vi "Power Rider Demo .vi"() -> ()   [LabVIEW 2017]
panel:
  out "Current [A]":sgl
  out "Vout [V]":sgl
  out "Switch":bool
  out "Status":u8(ring) items=["OFF", "ON", "ERROR", "FOREVER OFF"]
  out "Vin [V]":sgl
  out "Trip Type":u16(ring)=2 items=["Not tripped", "SW Tripped", "Hard Short", "MAX SW Tripped"]
  in  "ChannelNum":i32=1
  out "Unit P_N":string
  out "SW Version":string
  in  "dstAdd":u8=16
  in  "ID address":u8=85
  out "dllVersion":string
  # "Power Rider Demo"
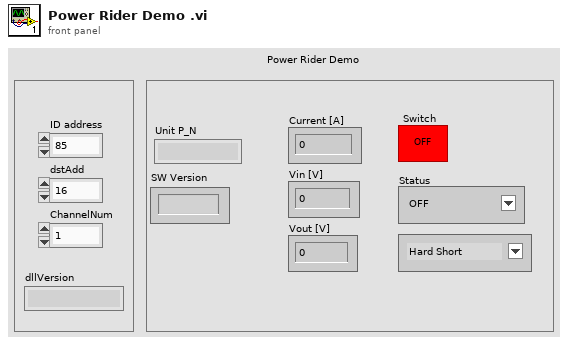
[diagram p1: front panel]
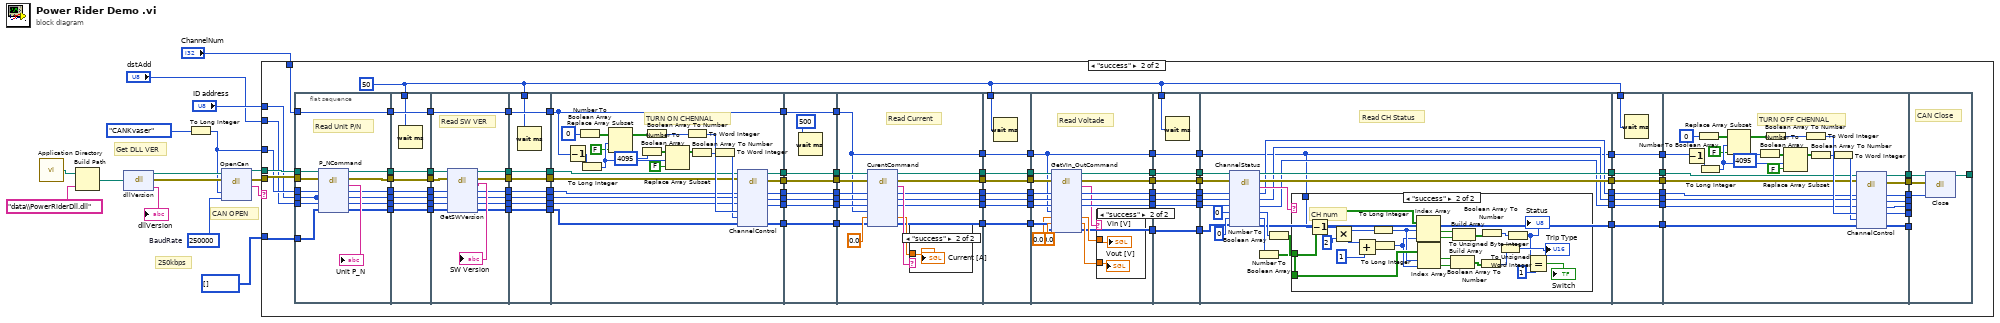
[diagram p0: block diagram]
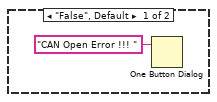
[diagram p2: hidden frame]
diagram:
  w12 = u32 250000  # BaudRate
  # "CAN OPEN"
  # "Get DLL VER"
  # "250kbps"
  n1 = call <vilib>:"Application Directory.vi"() -> ("Application Directory"=w16:path)
  n2 = Build Path(base path=w16, name or relative path="data\\PowerRiderDll.dll") -> (appended path=w14:path)
  n3 = dll-call lib="C:/Projects/Fuse/PowerRider-DLL-GUI/PRDLL/Labview/data/PowerRiderDll.dll" fn="dllVersion"(path in=w14) -> (path out=w11:path, error out=w10:errorcluster, "return type"=→"dllVersion":string)  [unwired: 2 in]
  n4 = To Long Integer(number=enum32{"None", "CANalystII", "UDP", "CANKvaser"}."CANKvaser") -> (32bit integer=w5:i32)
  n5 = dll-call lib="C:/Projects/Fuse/PowerRider-DLL-GUI/PRDLL/Labview/data/PowerRiderDll.dll" fn="OpenCan"(path in=w11, error in=w10, "type"=w5, "BaudRate"=w12) -> (path out=w9:path, error out=w8:errorcluster, "return type"=w7:string)  [unwired: 3 in]
  n6 = case shown="\"success\"" w7 {
    tunnel: w9 -> [_ w111]
    tunnel: w8 -> [_ w110]
    tunnel: w5 -> [_ w109]
    tunnel: "ID address" -> [_ w108]
    tunnel: "dstAdd" -> [_ w107]
    tunnel: u8[] [] ("PsNetwork") -> [_ w112]
    tunnel: "ChannelNum" -> [_ w106]
    frame "False", Default {
      n7 = One Button Dialog(message="CAN Open Error !!! ") -> ()  [unwired: 1 in, 1 out]
    }
    frame "success" {
      w18 = u32 50 ("milliseconds to wait")
      n8 = flat-sequence {
        tunnel: w106 -> [w130]
        tunnel: [w130] -> w113
        tunnel: w112 -> [w128]
        tunnel: w111 -> [w127]
        tunnel: w110 -> [w126]
        tunnel: w109 -> [w125]
        tunnel: [w124] -> _
        tunnel: w108 -> [w124]
        tunnel: w107 -> [w123]
        tunnel: [w122] -> w104
        tunnel: [w121] -> w102
        tunnel: [w120] -> w100
        tunnel: [w119] -> w98
        tunnel: [w118] -> w96
        tunnel: [w117] -> w94
        tunnel: [w138] -> w114
        tunnel: w113 -> [w138]
        tunnel: w18 -> [w137]
        tunnel: [w136] -> w105
        tunnel: w104 -> [w136]
        tunnel: [w135] -> w103
        tunnel: w102 -> [w135]
        tunnel: [w134] -> w101
        tunnel: w100 -> [w134]
        tunnel: [w133] -> w99
        tunnel: w98 -> [w133]
        tunnel: [w132] -> w97
        tunnel: w96 -> [w132]
        tunnel: [w131] -> w95
        tunnel: w94 -> [w131]
        tunnel: [w152] -> w93
        tunnel: w114 -> [w152]
        tunnel: w105 -> [w150]
        tunnel: w103 -> [w149]
        tunnel: w101 -> [w148]
        tunnel: w99 -> [w147]
        tunnel: w97 -> [w146]
        tunnel: w95 -> [w145]
        tunnel: [w144] -> w91
        tunnel: [w143] -> w89
        tunnel: [w142] -> w87
        tunnel: [w141] -> w85
        tunnel: [w140] -> w83
        tunnel: [w139] -> w81
        tunnel: w93 -> [w160]
        tunnel: [w160] -> w92
        tunnel: w91 -> [w159]
        tunnel: [w159] -> w90
        tunnel: w89 -> [w158]
        tunnel: [w158] -> w88
        tunnel: w87 -> [w157]
        tunnel: [w157] -> w86
        tunnel: w85 -> [w156]
        tunnel: [w156] -> w84
        tunnel: w83 -> [w155]
        tunnel: [w155] -> w82
        tunnel: w81 -> [w154]
        tunnel: [w154] -> w80
        tunnel: w18 -> [w153]
        tunnel: [w174] -> w115
        tunnel: w92 -> [w174]
        tunnel: w90 -> [w173]
        tunnel: w88 -> [w172]
        tunnel: w86 -> [w171]
        tunnel: w84 -> [w170]
        tunnel: w82 -> [w169]
        tunnel: w80 -> [w168]
        tunnel: [w167] -> w78
        tunnel: [w166] -> w76
        tunnel: [w165] -> w74
        tunnel: [w164] -> w72
        tunnel: [w163] -> w70
        tunnel: [w162] -> w68
        tunnel: [w195] -> w116
        tunnel: w115 -> [w195]
        tunnel: [w193] -> w79
        tunnel: w78 -> [w193]
        tunnel: [w192] -> w77
        tunnel: w76 -> [w192]
        tunnel: [w191] -> w75
        tunnel: w74 -> [w191]
        tunnel: [w190] -> w73
        tunnel: w72 -> [w190]
        tunnel: [w189] -> w71
        tunnel: w70 -> [w189]
        tunnel: [w188] -> w69
        tunnel: w68 -> [w188]
        tunnel: [w208] -> w67
        tunnel: [w207] -> w65
        tunnel: [w206] -> w63
        tunnel: [w205] -> w61
        tunnel: [w204] -> w58
        tunnel: w116 -> [w197]
        tunnel: w79 -> [w203]
        tunnel: w77 -> [w202]
        tunnel: w75 -> [w201]
        tunnel: w73 -> [w200]
        tunnel: w71 -> [w199]
        tunnel: w69 -> [w198]
        tunnel: [w197] -> w55
        tunnel: [w196] -> w54
        tunnel: w67 -> [w220]
        tunnel: [w220] -> w66
        tunnel: w65 -> [w219]
        tunnel: [w219] -> w64
        tunnel: w63 -> [w218]
        tunnel: [w218] -> w62
        tunnel: w61 -> [w214]
        tunnel: [w214] -> w60
        tunnel: [w213] -> w59
        tunnel: w58 -> [w217]
        tunnel: [w217] -> w57
        tunnel: w18 -> [w216]
        tunnel: [w215] -> w56
        tunnel: w55 -> [w215]
        tunnel: w54 -> [w213]
        tunnel: w66 -> [w236]
        tunnel: w64 -> [w235]
        tunnel: w62 -> [w234]
        tunnel: w60 -> [w232]
        tunnel: w59 -> [w231]
        tunnel: w57 -> [w237]
        tunnel: w56 -> [w221]
        tunnel: [w230] -> w53
        tunnel: [w229] -> w52
        tunnel: [w228] -> w51
        tunnel: [w227] -> w50
        tunnel: [w226] -> w49
        tunnel: [w222] -> w48
        tunnel: [w221] -> w29
        tunnel: w53 -> [w248]
        tunnel: w52 -> [w247]
        tunnel: w51 -> [w246]
        tunnel: w50 -> [w245]
        tunnel: w49 -> [w244]
        tunnel: w48 -> [w243]
        tunnel: w18 -> [w242]
        tunnel: [w248] -> w47
        tunnel: [w247] -> w46
        tunnel: [w246] -> w45
        tunnel: [w245] -> w44
        tunnel: [w244] -> w43
        tunnel: [w243] -> w42
        tunnel: w29 -> [w241]
        tunnel: [w241] -> w28
        tunnel: w47 -> [w263]
        tunnel: w46 -> [w264]
        tunnel: w45 -> [w261]
        tunnel: w44 -> [w260]
        tunnel: w43 -> [w259]
        tunnel: w42 -> [w262]
        tunnel: [w254] -> w41
        tunnel: [w255] -> w40
        tunnel: [w253] -> w39
        tunnel: [w252] -> w38
        tunnel: [w251] -> w37
        tunnel: [w250] -> w36
        tunnel: w28 -> [w249]
        tunnel: [w249] -> w20
        tunnel: w41 -> [w298]
        tunnel: w40 -> [w297]
        tunnel: w39 -> [w296]
        tunnel: w38 -> [w295]
        tunnel: w37 -> [w294]
        tunnel: w36 -> [w293]
        tunnel: w18 -> [w292]
        tunnel: [w298] -> w35
        tunnel: [w297] -> w34
        tunnel: [w296] -> w33
        tunnel: [w295] -> w32
        tunnel: [w294] -> w31
        tunnel: [w293] -> w30
        tunnel: w20 -> [w291]
        tunnel: [w291] -> w19
        tunnel: w35 -> [w312]
        tunnel: w34 -> [w313]
        tunnel: w33 -> [w311]
        tunnel: w32 -> [w310]
        tunnel: w31 -> [w309]
        tunnel: w30 -> [w308]
        tunnel: [w307] -> w27
        tunnel: [w306] -> w26
        tunnel: [w305] -> w25
        tunnel: [w304] -> w24
        tunnel: [w303] -> w23
        tunnel: [w302] -> w22
        tunnel: [w301] -> w21
        tunnel: w19 -> [w300]
        tunnel: w27 -> [w329]
        tunnel: w26 -> [w328]
        tunnel: w25 -> [_]
        tunnel: w24 -> [w330]
        tunnel: w23 -> [_]
        tunnel: w22 -> [_]
        tunnel: w21 -> [_]
        tunnel: [w327] -> _
        frame #0 {
          # "Read Unit P/N"
          n9 = dll-call lib="C:/Projects/Fuse/PowerRider-DLL-GUI/PRDLL/Labview/data/PowerRiderDll.dll" fn="P_NCommand"(path in=w127, error in=w126, "type"=w125, "ID"=w124, "dstAdd"=w123, "PsNetwork"=w128) -> (path out=w122:path, error out=w121:errorcluster, "return type"=→"Unit P_N":string, "type"=w120:i32, "ID"=w119:u8, "dstAdd"=w118:u8, "PsNetwork"=w117:u8[])  [unwired: 1 in]
        }
        frame #1 {
          n10 = Wait (ms)(milliseconds to wait=w137) -> ()  [unwired: 1 out]
        }
        frame #2 {
          # "Read SW VER"
          n11 = dll-call lib="C:/Projects/Fuse/PowerRider-DLL-GUI/PRDLL/Labview/data/PowerRiderDll.dll" fn="GetSWVersion"(path in=w150, error in=w149, "type"=w148, "ID"=w147, "dstAdd"=w146, "pSockAdd"=w145) -> (path out=w144:path, error out=w143:errorcluster, "return type"=→"SW Version":string, "type"=w142:i32, "ID"=w141:u8, "dstAdd"=w140:u8, "pSockAdd"=w139:u8[])  [unwired: 1 in]
        }
        frame #3 {
          n12 = Wait (ms)(milliseconds to wait=w153) -> ()  [unwired: 1 out]
        }
        frame #4 {
          # "TURN ON CHENNAL"
          n13 = Decrement(x=w174) -> (x-1=w181:i32)
          n14 = Number To Boolean Array(number=u16 0 ("element")) -> (Boolean array=w178:bool[])
          n15 = To Long Integer(number=w181) -> (32bit integer=w187:i32)
          n16 = Replace Array Subset(array=w178, new element=FALSE ("new element/subarray"), index=w187) -> (w179:bool[])
          n17 = Number To Boolean Array(number=u16 4095 ("mask")) -> (Boolean array=w182:bool[])
          n18 = Boolean Array To Number(Boolean array=w179) -> (number=w180:u32)
          n19 = Replace Array Subset(array=w182, new element=FALSE ("new element/subarray"), index=w187) -> (w183:bool[])
          n20 = To Word Integer(number=w180) -> (16bit integer=w186:i16)
          n21 = Boolean Array To Number(Boolean array=w183) -> (number=w184:u32)
          n22 = To Word Integer(number=w184) -> (16bit integer=w185:i16)
          n23 = dll-call lib="C:/Projects/Fuse/PowerRider-DLL-GUI/PRDLL/Labview/data/PowerRiderDll.dll" fn="ChannelControl"(path in=w173, error in=w172, "type"=w171, "ID"=w170, "dstAdd"=w169, "Conrol"=w186, "mask"=w185, "PSockAdd"=w168) -> (path out=w167:path, error out=w166:errorcluster, "type"=w165:i32, "ID"=w164:u8, "dstAdd"=w163:u16, "PSockAdd"=w162:u8[])  [unwired: 4 in]
        }
        frame #5 {
          n24 = Wait (ms)(milliseconds to wait=u32 500) -> ()  [unwired: 1 out]
        }
        frame #6 {
          # "Read Current"
          n25 = dll-call lib="C:/Projects/Fuse/PowerRider-DLL-GUI/PRDLL/Labview/data/PowerRiderDll.dll" fn="CurentCommand"(path in=w203, error in=w202, "type"=w201, "ID"=w200, "dstAdd"=w199, "Chan"=w197, "valcurr"=sgl 0.0, "PSockAdd"=w198) -> (path out=w208:path, error out=w207:errorcluster, "return type"=w210:string, "type"=w206:i32, "ID"=w205:u8, "dstAdd"=w196:u8, "valcurr"=w209:sgl, "PSockAdd"=w204:u8[])  [unwired: 2 in]
          n26 = case shown="\"success\"" w210 {
            tunnel: w209 -> [_ w212]
            frame "False", Default {
            }
            frame "success" {
              "Current [A]" <- w212
            }
          }
        }
        frame #7 {
          n27 = Wait (ms)(milliseconds to wait=w216) -> ()  [unwired: 1 out]
        }
        frame #8 {
          # "Read Voltade"
          n28 = dll-call lib="C:/Projects/Fuse/PowerRider-DLL-GUI/PRDLL/Labview/data/PowerRiderDll.dll" fn="GetVIn_OutCommand"(path in=w236, error in=w235, "type"=w234, "ID"=w232, "dstAdd"=w231, "ChannelNo"=w221, "vin"=sgl 0.0, "vou"=sgl 0.0, "PSockAdd"=w237) -> (path out=w229:path, error out=w230:errorcluster, "return type"=w225:string, "type"=w228:i32, "ID"=w227:u8, "dstAdd"=w226:u8, "vin"=w223:sgl, "vou"=w224:sgl, "PSockAdd"=w222:u8[])  [unwired: 2 in]
          n29 = case shown="\"success\"" w225 {
            tunnel: w224 -> [_ w240]
            tunnel: w223 -> [_ w239]
            frame "False", Default {
            }
            frame "success" {
              "Vin [V]" <- w239
              "Vout [V]" <- w240
            }
          }
        }
        frame #9 {
          n30 = Wait (ms)(milliseconds to wait=w242) -> ()  [unwired: 1 out]
        }
        frame #10 {
          # "Read CH Status"
          n31 = dll-call lib="C:/Projects/Fuse/PowerRider-DLL-GUI/PRDLL/Labview/data/PowerRiderDll.dll" fn="ChannelStatus"(path in=w264, error in=w263, "type"=w261, "ID"=w260, "dstAdd"=w259, "ChannelStat"=0, "ChannelTrip"=0, "PSockAdd"=w262) -> (path out=w255:path, error out=w254:errorcluster, "return type"=w258:string, "type"=w253:i32, "ID"=w252:u8, "dstAdd"=w251:u8, "ChannelStat"=w267:i32, "ChannelTrip"=w268:i32, "PSockAdd"=w250:u8[])  [unwired: 1 in]
          n32 = Number To Boolean Array(number=w268) -> (Boolean array=w256:bool[])
          n33 = Number To Boolean Array(number=w267) -> (Boolean array=w257:bool[])
          n34 = case shown="\"success\"" w258 {
            tunnel: w257 -> [_ w290]
            tunnel: w256 -> [_ w289]
            tunnel: w249 -> [_ w272]
            frame "False", Default {
            }
            frame "success" {
              # "CH num"
              n35 = Decrement(x=w272) -> (x-1=w274:i32)
              n36 = Multiply(x=w274, y=u8 2) -> (x*y=w286:i32)
              n37 = Add(x=w286, y=u8 1) -> (x+y=w285:i32)
              n38 = To Long Integer(number=w286) -> (32bit integer=w284:i32)
              n39 = To Long Integer(number=w285) -> (32bit integer=w283:i32)
              n40 = Index Array(array=w290, index #1=w284, index #2=w283) -> (element #1=w282:bool, element #2=w281:bool)
              n41 = Index Array(array=w289, index #1=w284, index #2=w283) -> (element #1=w279:bool, element #2=w280:bool)
              n42 = Build Array(w279, w280) -> (w277:bool[])
              n43 = Build Array(w282, w281) -> (w278:bool[])
              n44 = Boolean Array To Number(Boolean array=w277) -> (number=w275:u32)
              n45 = Boolean Array To Number(Boolean array=w278) -> (number=w276:u32)
              n46 = To Unsigned Word Integer(number=w275) -> (unsigned 16bit integer=→"Trip Type":u16)
              n47 = To Unsigned Byte Integer(number=w276) -> (unsigned 8bit integer=w269:u8)
              "Status" <- w269
              n48 = Equal?(x=w269, y=u8 1) -> (x = y?=→"Switch":bool)
            }
          }
        }
        frame #11 {
          n49 = Wait (ms)(milliseconds to wait=w292) -> ()  [unwired: 1 out]
        }
        frame #12 {
          # "TURN OFF CHENNAL"
          n50 = Decrement(x=w300) -> (x-1=w320:i32)
          n51 = Number To Boolean Array(number=u16 0 ("element")) -> (Boolean array=w317:bool[])
          n52 = To Long Integer(number=w320) -> (32bit integer=w326:i32)
          n53 = Replace Array Subset(array=w317, new element=FALSE ("new element/subarray"), index=w326) -> (w318:bool[])
          n54 = Number To Boolean Array(number=u16 4095 ("mask")) -> (Boolean array=w321:bool[])
          n55 = Boolean Array To Number(Boolean array=w318) -> (number=w319:u32)
          n56 = Replace Array Subset(array=w321, new element=FALSE ("new element/subarray"), index=w326) -> (w322:bool[])
          n57 = To Word Integer(number=w319) -> (16bit integer=w325:i16)
          n58 = Boolean Array To Number(Boolean array=w322) -> (number=w323:u32)
          n59 = To Word Integer(number=w323) -> (16bit integer=w324:i16)
          n60 = dll-call lib="C:/Projects/Fuse/PowerRider-DLL-GUI/PRDLL/Labview/data/PowerRiderDll.dll" fn="ChannelControl"(path in=w313, error in=w312, "type"=w311, "ID"=w310, "dstAdd"=w309, "Conrol"=w325, "mask"=w324, "PSockAdd"=w308) -> (path out=w307:path, error out=w304:errorcluster, "type"=w306:i32, "ID"=w305:u8, "dstAdd"=w303:u16, "Conrol"=w302:i16, "PSockAdd"=w301:u8[])  [unwired: 3 in]
        }
        frame #13 {
          # "CAN Close"
          n61 = dll-call lib="C:/Projects/Fuse/PowerRider-DLL-GUI/PRDLL/Labview/data/PowerRiderDll.dll" fn="Close"(path in=w329, error in=w330, "type"=w328) -> (path out=w327:path)  [unwired: 3 in, 1 out]
        }
      }
    }
  }
